vi "ScoreTracker(SubVI).vi"(8 "Elapsed Time":dbl, 9 "Score Array":i16[](array[numeric]), 10 "Numeric in":i32, 11 "Numeric 3":i16) -> (0 "LCD Bottom":string, 1 "LCD Top":string, 3 "Numeric out":i32)   [LabVIEW 2017]
panel:
  out "Add Ready?":bool
  out "error out":errorcluster
  in  "error in (no error)":errorcluster
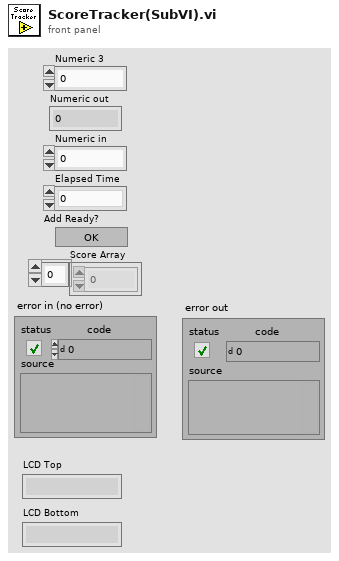
[diagram p1: front panel]
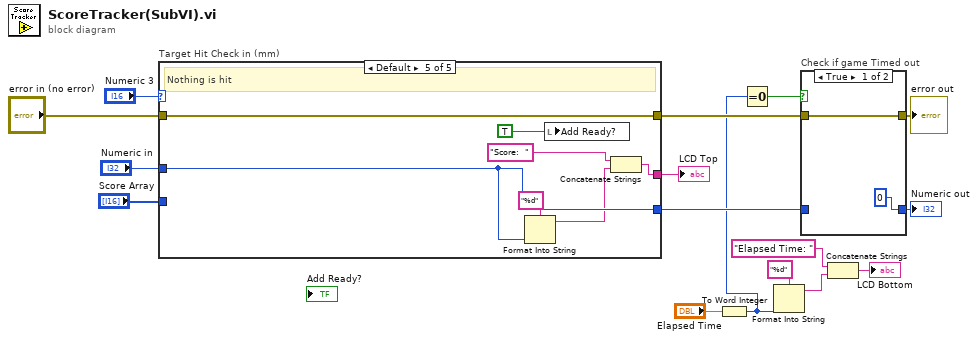
[diagram p0: block diagram]
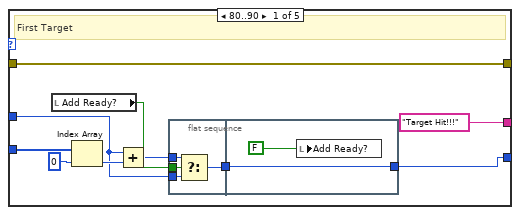
[diagram p3: hidden frame]
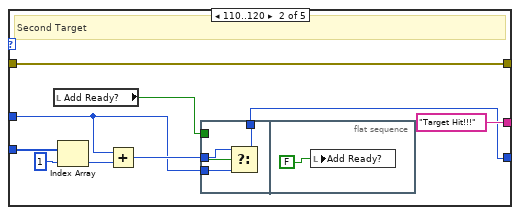
[diagram p4: hidden frame]
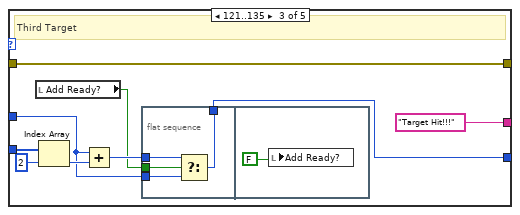
[diagram p5: hidden frame]
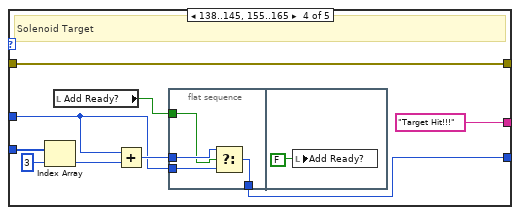
[diagram p6: hidden frame]
diagram:
  n1 = case "Target Hit Check in (mm)" shown="Default" "Numeric 3" {
    tunnel: [w17 w33 w47 w61 w77] -> w7
    tunnel: "Numeric in" -> [w19 w35 w49 w63 w77]
    tunnel: "Score Array" -> [w26 w41 w55 w69 _]
    tunnel: "error in (no error)" -> [w23 w38 w52 w66 w81]
    tunnel: [w23 w38 w52 w66 w81] -> w12
    tunnel: ["Target Hit!!!" "Target Hit!!!" "Target Hit!!!" "Target Hit!!!" w79] -> w8
    frame 80..90 {
      # "First Target"
      n2 = local read "Add Ready?"() -> (w21:bool)
      n3 = Index Array(array=w26, index=0) -> (element=w24:i16)
      n4 = Add(x=w19, y=w24) -> (x+y=w20:i32)
      n5 = flat-sequence {
        tunnel: w21 -> [w30]
        tunnel: w20 -> [w29]
        tunnel: w19 -> [w28]
        tunnel: [w27] -> w18
        tunnel: [w32] -> w17
        tunnel: w18 -> [w32]
        frame #0 {
          n6 = Select(t=w29, s=w30, f=w28) -> (s? t:f=w27:i32)
        }
        frame #1 {
          n7 = local write "Add Ready?"(FALSE) -> ()
        }
      }
    }
    frame 110..120 {
      # "Second Target"
      n8 = local read "Add Ready?"() -> (w34:bool)
      n9 = Index Array(array=w41, index=1) -> (element=w39:i16)
      n10 = Add(x=w35, y=w39) -> (x+y=w36:i32)
      n11 = flat-sequence {
        tunnel: w36 -> [w45]
        tunnel: w35 -> [w44]
        tunnel: w34 -> [w43]
        tunnel: [w42] -> w33
        frame #0 {
          n12 = Select(t=w45, s=w43, f=w44) -> (s? t:f=w42:i32)
        }
        frame #1 {
          n13 = local write "Add Ready?"(FALSE) -> ()
        }
      }
    }
    frame 121..135 {
      # "Third Target"
      n14 = local read "Add Ready?"() -> (w48:bool)
      n15 = Index Array(array=w55, index=2) -> (element=w53:i16)
      n16 = Add(x=w49, y=w53) -> (x+y=w50:i32)
      n17 = flat-sequence {
        tunnel: w50 -> [w59]
        tunnel: w49 -> [w58]
        tunnel: w48 -> [w57]
        tunnel: [w56] -> w47
        frame #0 {
          n18 = Select(t=w59, s=w57, f=w58) -> (s? t:f=w56:i32)
        }
        frame #1 {
          n19 = local write "Add Ready?"(FALSE) -> ()
        }
      }
    }
    frame 138..145, 155..165 {
      # "Solenoid Target"
      n20 = Index Array(array=w69, index=3) -> (element=w67:i16)
      n21 = local read "Add Ready?"() -> (w62:bool)
      n22 = Add(x=w63, y=w67) -> (x+y=w64:i32)
      n23 = flat-sequence {
        tunnel: w64 -> [w73]
        tunnel: w63 -> [w72]
        tunnel: w62 -> [w71]
        tunnel: [w70] -> w61
        frame #0 {
          n24 = Select(t=w73, s=w71, f=w72) -> (s? t:f=w70:i32)
        }
        frame #1 {
          n25 = local write "Add Ready?"(FALSE) -> ()
        }
      }
    }
    frame Default {
      # "Nothing is hit"
      n26 = Format Into String(format string="%d", w77) -> (resulting string=w76:string)  [unwired: 2 in, 1 out]
      n27 = local write "Add Ready?"(TRUE) -> ()
      n28 = Concatenate Strings("Score:  ", w76) -> (w79:string)
    }
  }
  "LCD Top" <- w8
  n29 = To Word Integer(number="Elapsed Time") -> (16bit integer=w1:i16)
  n30 = Equal To 0?(x=w1) -> (x = 0?=w2:bool)
  n31 = Format Into String(format string="%d", w1) -> (resulting string=w4:string)  [unwired: 2 in, 1 out]
  n32 = case "Check if game Timed out" shown="True" w2 {
    tunnel: w12 -> [w83 w85]
    tunnel: [w83 w85] -> w11
    tunnel: w7 -> [_ w84]
    tunnel: [0 w84] -> w6
    frame True {
    }
    frame False {
    }
  }
  "Numeric out" <- w6
  "error out" <- w11
  n33 = Concatenate Strings("Elapsed Time: ", w4) -> (→"LCD Bottom":string)
